vi "testIntStringToInt.vi"(8 "error in (no error)":errorcluster, 11 "TestCase in":refnum<class "UnitTestIntClass.lvclass">) -> (0 "error out":errorcluster, 3 "TestCase out":refnum<class "UnitTestIntClass.lvclass">)   [LabVIEW 2011, in "UnitTestIntClass.lvclass"]
uses:
  UnitTestIntClass.lvclass
  <vilib>/addons/_JKI Toolkits/VI Tester/TestCase.llb/TestCase.lvclass
  IntClass/IntClass.lvclass
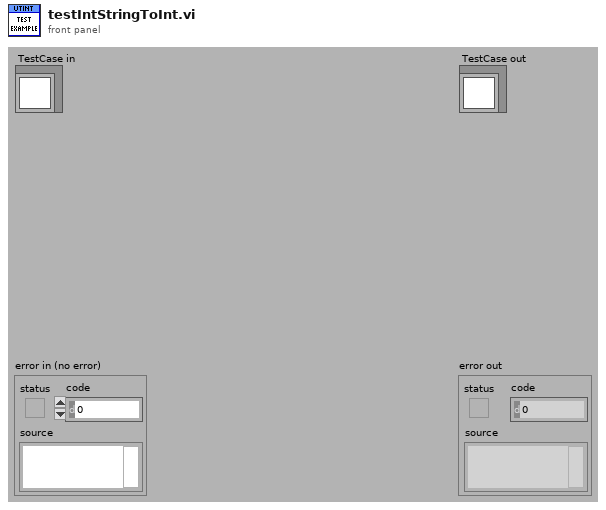
[diagram p1: front panel]
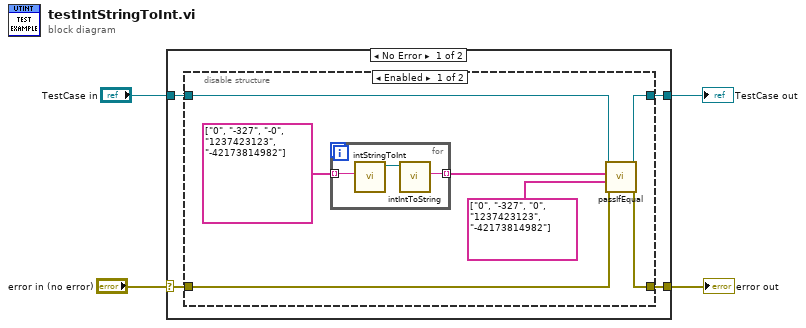
[diagram p0: block diagram]
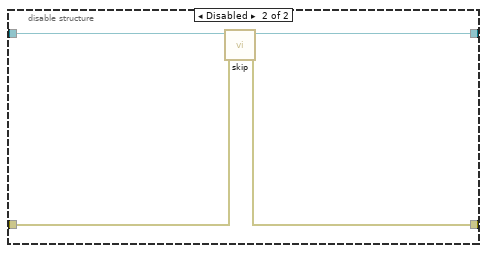
[diagram p2: hidden frame]
diagram:
  n1 = case shown="No Error" "error in (no error)" {
    selector: "error in (no error)" -> [w6 w24]
    tunnel: [w5 w24] -> w3
    tunnel: [w7 w23] -> w1
    tunnel: "TestCase in" -> [w8 w23]
    frame No Error {
      n2 = disable-structure shown="Enabled" {
        disable-tunnel: w8 -> [w12 w22]
        disable-tunnel: [w15 w19] -> w7
        disable-tunnel: w6 -> [w14 w21]
        disable-tunnel: [w13 w20] -> w5
        frame Enabled {
          n3 = for {
            tunnel: string[] ["0", "-327", "-0", "1237423123", "-42173814982"] -> [w18] mode=indexing
            tunnel: [w16] -> w9 mode=indexing
            n4 = call "intStringToInt.vi"("String in"=w18) -> ("Int out"=w17:refnum<class "IntClass.lvclass">)  [unwired: 9 in, 1 out]
            n5 = call "intIntToString.vi"("Int in"=w17) -> ("String"=w16:string)  [unwired: 7 in, 3 out]
          }
          n6 = call-dynamic "passIfEqual.vi"("error in (no error)"=w14, "y"=string[] ["0", "-327", "0", "1237423123", "-42173814982"], "x"=w9, "TestCase in"=w12) -> ("error out"=w13:errorcluster, "TestCase out"=w15:refnum<class "UnitTestIntClass.lvclass">)  [unwired: 6 in]
        }
        frame Disabled {
          n7 = call <vilib>:"skip.vi"("error in (no error)"=w21, "TestCase in"=w22) -> ("error out"=w20:errorcluster, "TestCase out"=w19:refnum<class "UnitTestIntClass.lvclass">)  [unwired: 8 in]
        }
      }
    }
    frame Error {
    }
  }
  "error out" <- w3
  "TestCase out" <- w1
